vi "util-io-filter.vi"(10 "IO Search Conf":T3={"Device"=1, "Label"="myDout", "Type"=enum."DO", "Mode"=enum."RIO", "Tags"=""} {"Device" max=99 format="%02d"}, 11 "IO Configs List":T4[](array[typedef]) {"calibration"."Y" format="%#.3f"; "calibration"."X" format="%#.3f"; "ADDR" format="%04d"}) -> (3 "Search Results":T4[](array[typedef]) {"calibration"."Y" format="%#.3f"; "calibration"."X" format="%#.3f"; "ADDR" format="%04d"})   [LabVIEW 2024]
uses:
  controls/IONode.ctl
  controls/type.address.ctl
  controls/enum.io.type.ctl
  controls/enum.io.mode.ctl
  controls/typeXyPoint.ctl
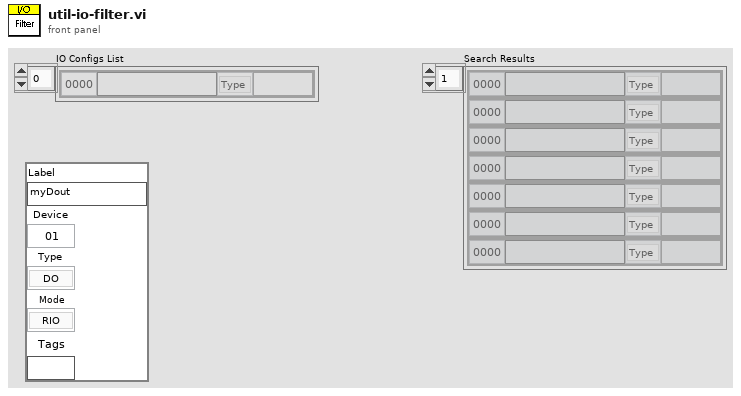
[diagram p1: front panel]
types:
  T1 = typedef "enum.io.type.ctl" = enum16{"Type", "DI", "DO", "AI", "AO", "VL", "BUF"}
  T2 = typedef "enum.io.mode.ctl" = enum16{"Mode", "RIO", "SIM"}
  T3 = cluster{"Device":u8, "Label":string, "Type":T1, "Mode":T2, "Tags":string}
  T4 = typedef "IONode.ctl" = cluster{"ADDR":T5, "Label":string, "Type":T1, "Mode":T2, "Value":string, "Tags":string, "calibration":T6[]}
  T5 = typedef "type.address.ctl" = u16
  T6 = typedef "typeXyPoint.ctl" = cluster{"X":dbl, "Y":dbl}
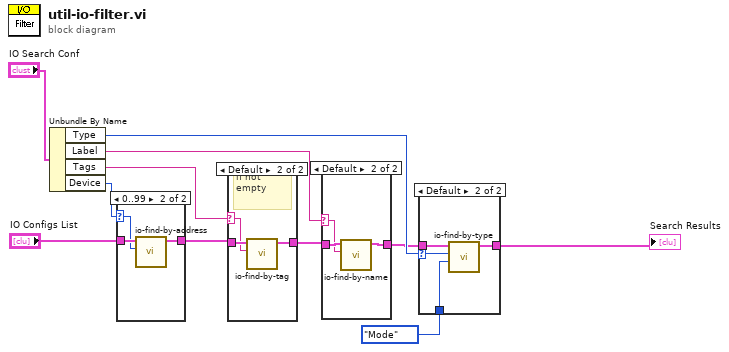
[diagram p0: block diagram]
diagram:
  n1 = Unbundle By Name("IO Search Conf") -> ("Type"=w10:T1, "Label"=w6:string, "Tags"=w5:string, "Device"=w2:u8)
  n2 = case shown="0..99" w2 {
    selector: w2 -> [_ w13]
    tunnel: "IO Configs List" -> [w12 w15]
    tunnel: [w12 w14] -> w4
    frame Default {
    }
    frame 0..99 {
      n3 = call "io-find-by-address.vi"("Device Address"=w13, "UiIoConfig"=w15) -> ("Array"=w14:T4[])  [unwired: 9 in]
    }
  }
  n4 = case shown="Default" w5 {
    selector: w5 -> [_ w17]
    tunnel: w4 -> [w16 w19]
    tunnel: [w16 w18] -> w7
    frame "" {
    }
    frame Default {
      # "if not empty"
      n5 = call "io-find-by-tag.vi"("Tag"=w17, "IOConfigs in"=w19) -> ("Filtered IOConfigs out"=w18:T4[])  [unwired: 9 in]
    }
  }
  n6 = case shown="Default" w6 {
    selector: w6 -> [_ w22]
    tunnel: w7 -> [w20 w23]
    tunnel: [w20 w21] -> w8
    frame "" {
    }
    frame Default {
      n7 = call "io-find-by-name.vi"("IO Name"=w22, "IO Nodes in"=w23) -> ("IO Nodes out"=w21:T4[])  [unwired: 7 in, 2 out]
    }
  }
  n8 = case shown="Default" w10 {
    selector: w10 -> [_ w26]
    tunnel: w8 -> [w24 w28]
    tunnel: [w24 w27] -> w9
    tunnel: enum.io.mode."Mode" ("Mode(Any)") -> [_ w25]
    frame "Type" {
    }
    frame Default {
      n9 = call "io-find-by-type.vi"("Mode(Any)"=w25, "Type"=w26, "IOConfigs in"=w28) -> ("Search Results"=w27:T4[])  [unwired: 8 in]
    }
  }
  "Search Results" <- w9
